vi "求最小公倍数.vi"(8 "n":i32, 11 "m":i32) -> (3 "lcm(m,n)":i32)   [LabVIEW 2011]
doc: "功能：\n\n利用最大公约数数计算整数m、n的最小公倍数数。\n\nCSXCS_366创建。"
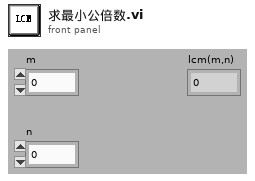
[diagram p1: front panel]
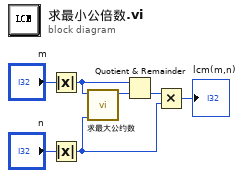
[diagram p0: block diagram]
diagram:
  n1 = Absolute Value(x="m") -> (abs(x)=w5:i32)
  n2 = Absolute Value(x="n") -> (abs(x)=w2:i32)
  n3 = call "求最大公约数.vi"("n"=w2, "m"=w5) -> ("gcd(m,n)"=w3:i32)  [unwired: 9 in]
  n4 = Quotient & Remainder(x=w5, y=w3) -> (floor(x/y)=w1:i32)  [unwired: 1 out]
  n5 = Multiply(x=w1, y=w2) -> (x*y=→"lcm(m,n)":i32)
